vi "Send Result Data_ZA.vi"(7 "Message Priority (Normal)":T2=enum."Normal", 8 "error in (no error)":errorcluster, 10 "ResultData":T1, 11 "Message Enqueuer":refnum<class "Message Enqueuer.lvclass">) -> (0 "error out":errorcluster, 3 "Message Enqueuer out":refnum<class "Message Enqueuer.lvclass">)   [LabVIEW 2015, in "Result Data_ZA Msg.lvclass"]
doc: "This VI sends the message to an actor."
uses:
  Result Data_ZA Msg.lvclass
  <vilib>/ActorFramework/Message Enqueuer/Message Enqueuer.lvclass
  <vilib>/ActorFramework/Message Enqueuer/Message Priority.ctl
  Zen Analytics/Dependency/GetData Cluster.ctl
  Zen Analytics/Zen Analytics.lvclass
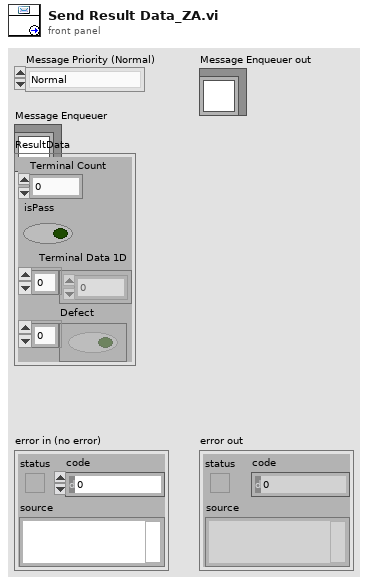
[diagram p1: front panel]
types:
  T1 = typedef "Zen Analytics.lvclass/GetData Cluster.ctl" = cluster{"Terminal Count":u32, "isPass":bool, "Terminal Data 1D":dbl[], "Defect":bool[]}
  T2 = typedef "Actor Framework.lvlib/Message Enqueuer.lvclass/Message Priority.ctl" = enum16{"Low", "Normal", "High"}
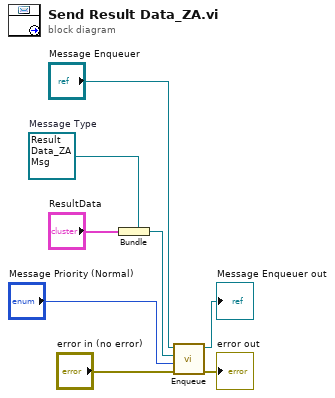
[diagram p0: block diagram]
diagram:
  w5 = refnum<class "Result Data_ZA Msg.lvclass"> refnum  # Message Type
  n1 = Bundle(cluster=w5, "ResultData") -> (w4:refnum<class "Result Data_ZA Msg.lvclass">)
  n2 = call <vilib>:"Enqueue.vi"("error in (no error)"="error in (no error)", "Message Priority (Normal)"="Message Priority (Normal)", "Message"=w4, "Message Enqueuer in"="Message Enqueuer") -> ("error out"=→"error out":errorcluster, "Message Enqueuer out"=→"Message Enqueuer out":refnum<class "Message Enqueuer.lvclass">)  [unwired: 6 in]
